vi "RemoveBadSpotImage-v3.vi"(4 "error in":errorcluster, 6 "ImgDataArray":T2(array[cluster]), 7 "Img Array In":T1[](array[typedef])) -> (0 "error out":errorcluster, 1 "Img Array Out":T1[](array[typedef]), 2 "Averages":T3={"Centroid Avg"={"X"=239.10901, "Y"=287.93375}, "Max Intensity Avg"=0.0, "Radius Avg"={"Rx"=239.10901, "Ry"=287.93375}}, 3 "Img Array Sorted":T1[](array[typedef]))   [LabVIEW 2013]
uses:
  <vilib>/vision/Image Controls.llb/IMAQ Image.ctl
panel:
  out "size(s)":i32
  out "result":bool
  out "counter":i32
  in  "Viewer":bool
  out "Image":T1(plugin-control)
  out "Numeric":i32
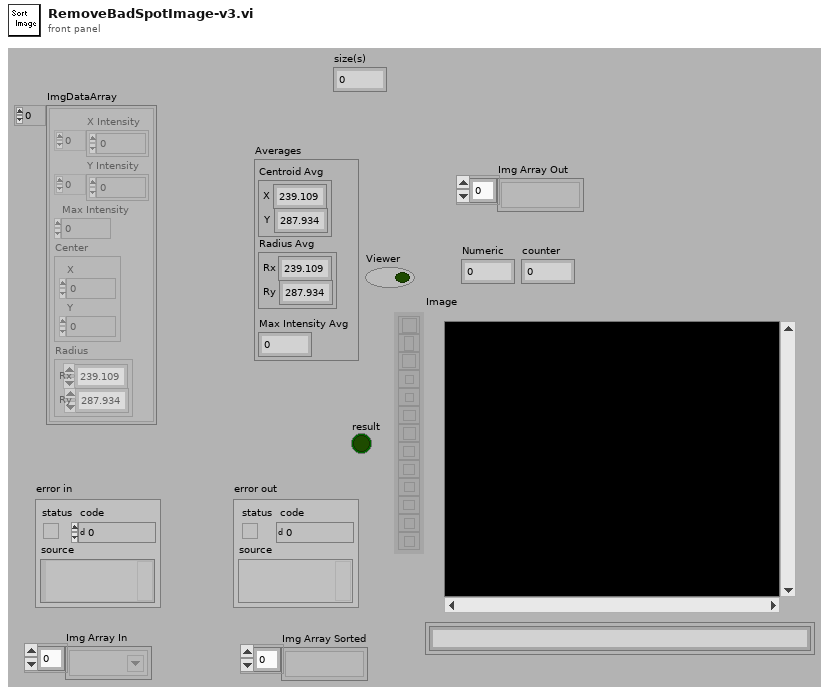
[diagram p1: front panel]
types:
  T1 = typedef "IMAQ Image.ctl" = refnum<image>
  T2 = cluster{"X Intensity":u8[], "Y Intensity":u8[], "Max Intensity":sgl, "Center":cluster{"X":sgl, "Y":sgl}, "Radius":cluster{"Rx":sgl, "Ry":sgl}}[]
  T3 = cluster{"Centroid Avg":cluster{"X":sgl, "Y":sgl}, "Max Intensity Avg":sgl, "Radius Avg":cluster{"Rx":sgl, "Ry":sgl}}
  T4 = typedef "Image Type" = u32
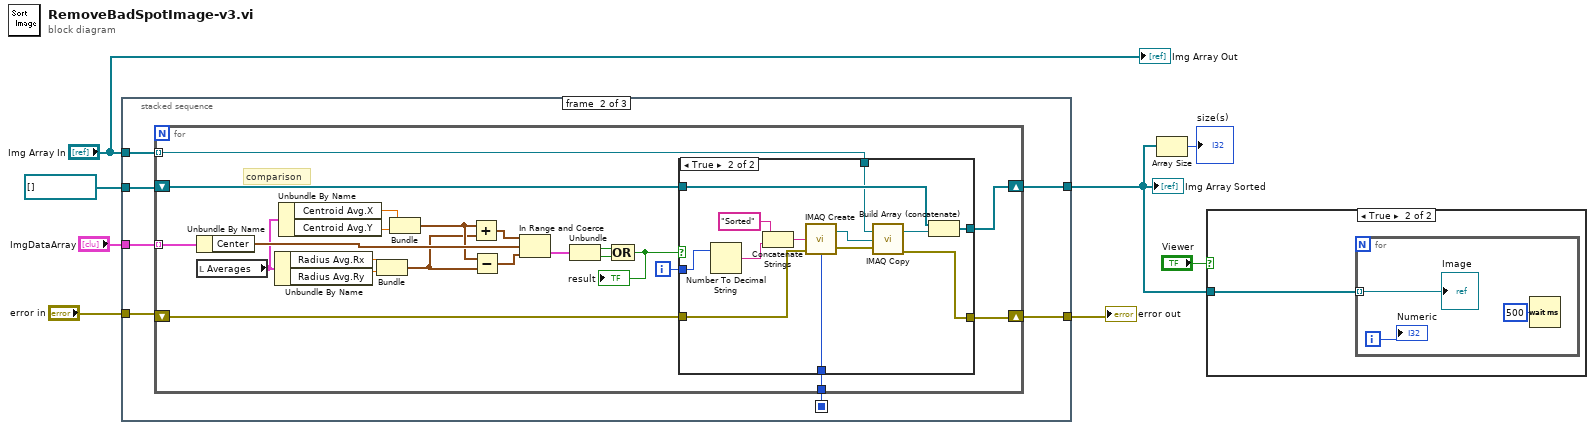
[diagram p0: block diagram]
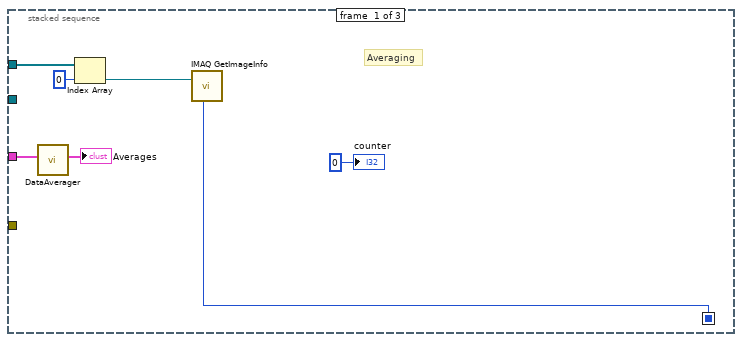
[diagram p2: hidden frame]
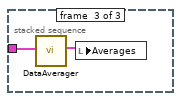
[diagram p4: hidden frame]
diagram:
  n1 = stacked-sequence {
    seq-local: [w9 _ _] -> [_ w16 _]
    tunnel: "ImgDataArray" -> [w14 w22 w61]
    tunnel: "Img Array In" -> [w12 w21 _]
    tunnel: [_ w18 _] -> w6
    tunnel: "error in" -> [_ w20 _]
    tunnel: [_ w19 _] -> w3
    tunnel: T1[] [] ("Img Array Sorted") -> [_ w17 _]
    frame #0 {
      # "Averaging"
      n2 = call "DataAverager.vi"("ImgDataArray"=w14) -> ("Averages"=→"Averages":T3)  [unwired: 6 out]
      n3 = Index Array(array=w12, index=0) -> (element=w11:T1)
      n4 = call "IMAQ GetImageInfo"("Image"=w11) -> ("Image Type"=w9:T4)  [unwired: 3 in, 7 out]
      "counter" <- 0
    }
    frame #1 {
      n5 = for {
        tunnel: w22 -> [w40] mode=indexing
        tunnel: w21 -> [w32] mode=indexing
        shift-right: [w26] -> w19
        shift-left: w20 -> [w27]
        shift-right: [w24] -> w18
        shift-left: w17 -> [w25]
        tunnel: w16 -> [w23]
        i -> [w31]
        # "comparison"
        n6 = Unbundle By Name(w40) -> ("Center"=w39:cluster{"X":sgl, "Y":sgl})
        n7 = local read "Averages"() -> (w36:T3)
        n8 = Unbundle By Name(w36) -> ("Radius Avg.Rx"=w38:sgl, "Radius Avg.Ry"=w37:sgl)
        n9 = Unbundle By Name(w36) -> ("Centroid Avg.X"=w35:sgl, "Centroid Avg.Y"=w34:sgl)
        n10 = Bundle("Rx"=w38, "Ry"=w37) -> (w28:cluster{"Rx":sgl, "Ry":sgl})  [unwired: 1 out]
        n11 = Bundle("X"=w35, "Y"=w34) -> (w29:cluster{"X":sgl, "Y":sgl})  [unwired: 1 out]
        n12 = Add(x=w29, y=w28) -> (x+y=w41:cluster{sgl, sgl})
        n13 = Subtract(x=w29, y=w28) -> (x-y=w33:cluster{sgl, sgl})
        n14 = In Range and Coerce(upper limit=w41, x=w39, lower limit=w33) -> (In Range?=w42:cluster{"X":bool, "Y":bool})  [unwired: 1 out]
        n15 = Unbundle(w42) -> ("X"=w43:bool, "Y"=w44:bool)
        n16 = Compound Arithmetic op=OR(w43, w44) -> (w30:bool)
        "result" <- w30
        n17 = case shown="True" w30 {
          tunnel: w31 -> [_ w57]
          tunnel: w32 -> [_ w49]
          tunnel: w27 -> [w46 w54]
          tunnel: [w46 w53] -> w26
          tunnel: w25 -> [w45 w51]
          tunnel: [w45 w50] -> w24
          tunnel: w23 -> [_ w47]
          frame False {
          }
          frame True {
            n18 = Number To Decimal String(number=w57) -> (decimal integer string=w56:string)  [unwired: 1 in]
            n19 = Concatenate Strings("Sorted", w56) -> (w58:string)
            n20 = call "IMAQ Create"("Image Name"=w58, "Image Type"=w47, "error in (no error)"=w54) -> ("New Image"=w48:T1, "error out"=w55:errorcluster)  [unwired: 2 in]
            n21 = call "IMAQ Copy"("error in (no error)"=w55, "Image Dst"=w48, "Image Src"=w49) -> ("error out"=w53:errorcluster, "Image Dst Out"=w52:T1)  [unwired: 3 in]
            n22 = Build Array (concatenate)(w51, w52) -> (w50:T1[])
          }
        }
      }
    }
    frame #2 {
      n23 = call "DataAverager.vi"("ImgDataArray"=w61) -> ("Averages"=w60:T3)  [unwired: 6 out]
      n24 = local write "Averages"(w60) -> ()
    }
  }
  "Img Array Sorted" <- w6
  "error out" <- w3
  n25 = Array Size(array=w6) -> (size(s)=→"size(s)":i32)
  n26 = case shown="True" "Viewer" {
    tunnel: w6 -> [_ w62]
    frame False {
    }
    frame True {
      n27 = for {
        tunnel: w62 -> [w63] mode=indexing
        i -> [w65]
        n28 = Wait (ms)(milliseconds to wait=u32 500 ("millisecond timer value")) -> ()  [unwired: 1 out]
        "Image" <- w63
        "Numeric" <- w65
      }
    }
  }
  "Img Array Out" <- "Img Array In"
